vi "Running Average.vi"(8 "Error In":errorcluster, 11 "Async State Vars 2":T1) -> (0 "Error Out":errorcluster, 3 "Async State Vars out":T1)   [LabVIEW 2015, in "Waveform-Processing-Custom-Device Shared.lvlib" / "Running Average.lvlib"]
uses:
  Shared/Running Average/Running Average.lvlib
  Types/AsyncStateVariables.ctl
  <vilib>/NI Veristand/Custom Device Waveform API/Single Waveform Read (DBL)/Single Waveform Read (DBL).lvclass
  <vilib>/NI Veristand/Custom Device Waveform API/Single Waveform Write (DBL)/Single Waveform Write (DBL).lvclass
  <vilib>/NI Veristand/Custom Device API/Waveform Data Reference.ctl
  <vilib>/NI/NIVS Inline Async API/_Data Access Engine/Data Access Engine/Types/Write.DVR.ctl
  <vilib>/NI/NIVS Inline Async API/_Data Access Engine/Access Type Classes/Write/Write.lvclass
  <vilib>/NI/NIVS Inline Async API/_Data Access Engine/Data Access Engine/Types/Read.DVR.ctl
  <vilib>/NI/NIVS Inline Async API/_Data Access Engine/Access Type Classes/Read/Read.lvclass
  <userlib>/Circular Buffer/Controls/Circular Buffer Operations.ctl
  <vilib>/NI/NIVS Inline Async API/_Data Access Engine/Access Type Classes/Read/Read.lvclass/Read.ctl
  <vilib>/NI/NIVS Inline Async API/_Data Access Engine/Access Type Classes/Write/Write.lvclass/Write.ctl
  <vilib>/NI/NIVS Inline Async API/_Data Access Engine/Data Access Engine/Methods/Read.Data.vi
  <vilib>/Analysis/baseanly.llb/Mean (DBL).vi
  <vilib>/NI/NIVS Inline Async API/_Data Access Engine/Data Access Engine/Methods/Write.Data.vi
  <vilib>/NI/NIVS Inline Async API/_Data Access Engine/Access Type Classes/Read/Read.ProcessData.vi
  <vilib>/NI/NIVS Inline Async API/_Data Access Engine/Access Type Classes/Write/Write.ProcessData.vi
  <userlib>/Circular Buffer/Instance VIs/Circular Buffer(2D DBL).vi
  <userlib>/Circular Buffer/Circular Buffer.lvlib
  <vilib>/Analysis/NI_AALBase.lvlib
  <vilib>/NI/NIVS Inline Async API/_Data Access Engine/Data Access Engine/Data Access Engine.lvclass
  Waveform-Processing-Custom-Device Engine.lvlib
  <vilib>/NI VeriStand/Custom Device API/Custom Device API.lvlib
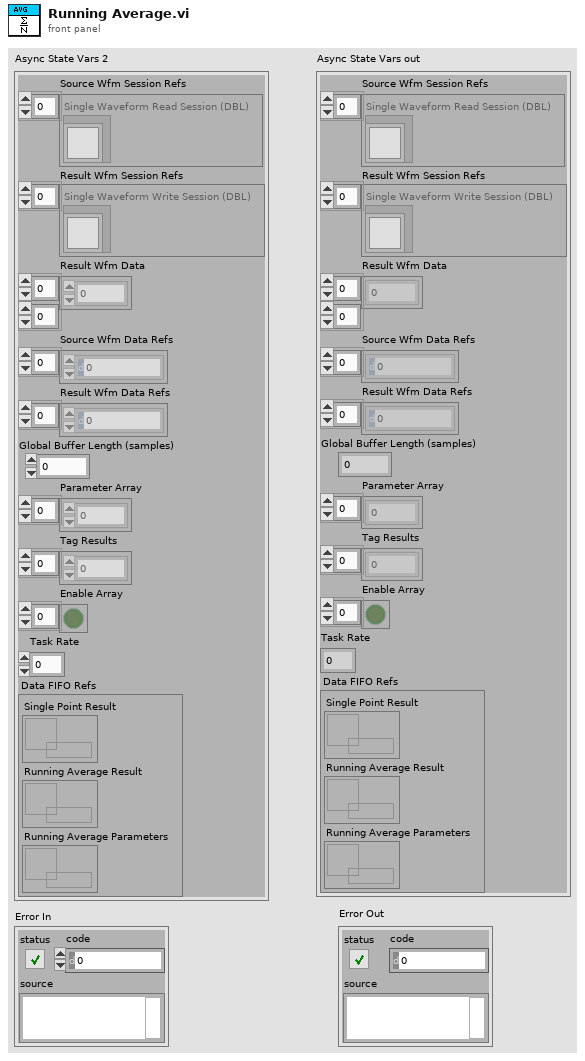
[diagram p1: front panel]
types:
  T1 = typedef "Waveform-Processing-Custom-Device Engine.lvlib/AsyncStateVariables.ctl" = cluster{"Source Wfm Session Refs":refnum<class "Single Waveform Read (DBL).lvclass">[], "Result Wfm Session Refs":refnum<class "Single Waveform Write (DBL).lvclass">[], "Result Wfm Data":dbl[][], "Source Wfm Data Refs":T2[], "Result Wfm Data Refs":T2[], "Global Buffer Length (samples)":dbl, "Parameter Array":dbl[], "Tag Results":dbl[], "Enable Array":bool[], "Task Rate":dbl, "Data FIFO Refs":cluster{"Single Point Result":T3, "Running Average Result":T3, "Running Average Parameters":T4}}
  T2 = typedef "Custom Device API.lvlib/Waveform Data Reference.ctl" = i32
  T3 = typedef "Data Access Engine.lvlib/Data Access Engine.lvclass/Write.DVR.ctl" = refnum<data-value>
  T4 = typedef "Data Access Engine.lvlib/Data Access Engine.lvclass/Read.DVR.ctl" = refnum<data-value>
  T5 = typedef "Circular Buffer.lvlib/Circular Buffer Operations.ctl" = enum16{"Initialize", "Get Backlog", "Write", "Read (continuous)", "Read (most recent)"}
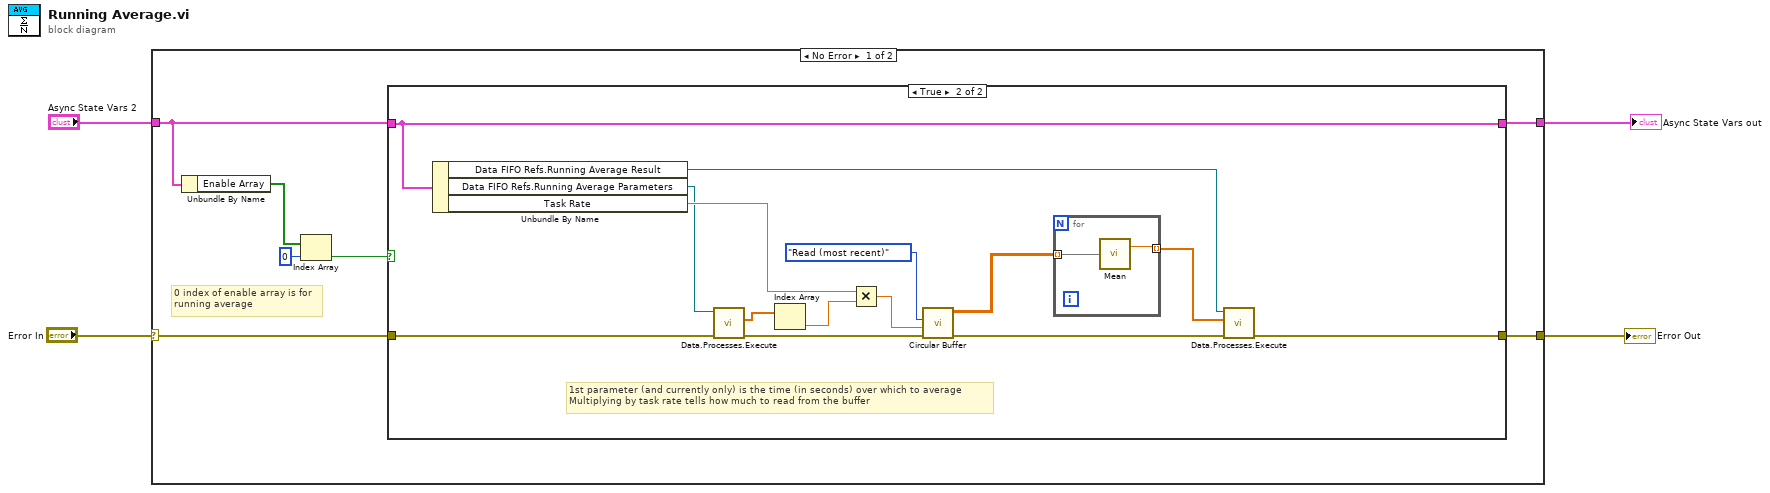
[diagram p0: block diagram]
diagram:
  n1 = case shown="No Error" "Error In" {
    selector: "Error In" -> [w11 w31]
    tunnel: [w10 w31] -> w3
    tunnel: "Async State Vars 2" -> [w8 w30]
    tunnel: [w9 w30] -> w1
    frame No Error {
      # "0 index of enable array is for\nrunning average"
      n2 = Unbundle By Name(w8) -> ("Enable Array"=w7:bool[])
      n3 = Index Array(array=w7, index=0) -> (element=w6:bool)
      n4 = case shown="True" w6 {
        tunnel: w11 -> [w13 w23]
        tunnel: [w13 w19] -> w10
        tunnel: w8 -> [w12 w25]
        tunnel: [w12 w25] -> w9
        frame False {
        }
        frame True {
          # "1st parameter (and currently only) is the time (in seconds) over which to average\nMultiplying by task rate tells how much to read from the buffer"
          n5 = Unbundle By Name(w25) -> ("Data FIFO Refs.Running Average Result"=w16:T3, "Data FIFO Refs.Running Average Parameters"=w17:T4, "Task Rate"=w18:dbl)
          n6 = call-poly <vilib>:"Data.Processes.Execute.vi"("error in (no error)"=w23, "Ref"=w17) -> ("error out"=w22:errorcluster, "Values"=w21:dbl[])  [unwired: 7 in, 1 out]
          n7 = Index Array(array=w21) -> (element=w14:dbl)  [unwired: 1 in]
          n8 = Multiply(x=w18, y=w14) -> (x*y=w24:dbl)
          n9 = call-poly <userlib>:"Circular Buffer.vi"("error in (no error)"=w22, "Read Size"=w24, "Operation"=Circular_Buffer_Operations."Read (most recent)") -> ("error out"=w20:errorcluster, "Data Out"=w26:dbl[][])  [unwired: 5 in, 2 out]
          n10 = for {
            tunnel: w26 -> [w29] mode=indexing
            tunnel: [w28] -> w15 mode=indexing
            n11 = call-poly <vilib>:"Mean.vi"("X"=w29) -> ("mean"=w28:dbl)  [unwired: 1 out]
          }
          n12 = call-poly <vilib>:"Data.Processes.Execute.vi"("error in (no error)"=w20, "Values"=w15, "Ref"=w16) -> ("error out"=w19:errorcluster)  [unwired: 8 in]
        }
      }
    }
    frame Error {
    }
  }
  "Error Out" <- w3
  "Async State Vars out" <- w1
